vi "midiinclose.vi"(4 "error in (no error)":errorcluster, 7 "hmidiin":i32) -> (0 "error out":errorcluster, 3 "output param":i32)   [LabVIEW 2014]
doc: "Closes the reference to the MIDI Input Device."
uses:
  mididll.dll
panel:
  # "Input Data"
  # "Local Data"
  # "Output Data"
  # "No local data."
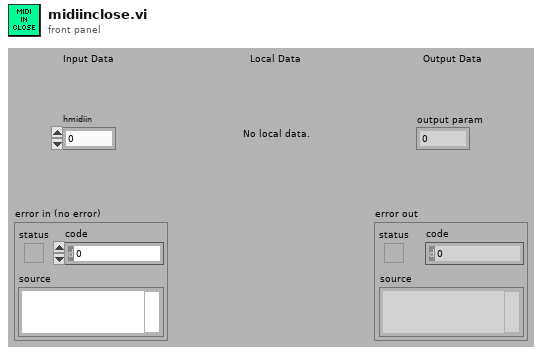
[diagram p1: front panel]
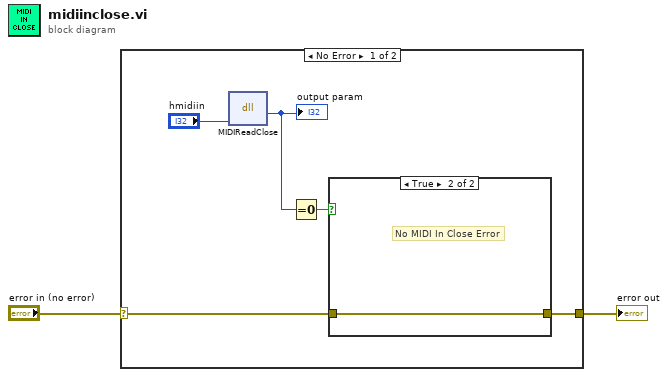
[diagram p0: block diagram]
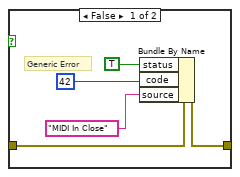
[diagram p2: hidden frame]
diagram:
  n1 = case shown="No Error" "error in (no error)" {
    selector: "error in (no error)" -> [w4 w14]
    tunnel: [w3 w14] -> w1
    frame No Error {
      n2 = dll-call lib="C:/Users/jag2k2/Desktop/Flashcards/MIDI Throughput Release 1.0/LabVIEW Code/MIDIDLL.dll" fn="MIDIReadClose"("hmidiin"="hmidiin") -> (w5:i32)  [unwired: 4 in, 2 out]
      "output param" <- w5
      n3 = Equal To 0?(x=w5) -> (x = 0?=w6:bool)
      n4 = case shown="True" w6 {
        tunnel: w4 -> [w12 w13]
        tunnel: [w11 w13] -> w3
        frame False {
          # "Generic Error"
          n5 = Bundle By Name(cluster=w12, "status"=TRUE, "code"=42, "source"="MIDI In Close") -> (w11:errorcluster)
        }
        frame True {
          # "No MIDI In Close Error"
        }
      }
    }
    frame Error {
    }
  }
  "error out" <- w1
